vi "Map Tags to Channels.vi"(7 "instance id":string, 8 "error in (no error)":errorcluster, 9 "String Array":string[][](array[string]), 10 "Lines":T1[](array[typedef]), 11 "engine configuration in":refnum<class "engine configuration.lvclass">) -> (0 "error out":errorcluster, 3 "engine configuration out":refnum<class "engine configuration.lvclass">)   [LabVIEW 2015, in "PID Module editor node.lvclass"]
uses:
  PID Module editor node.lvclass
  module/configuration/Line.ctl
  <vilib>/NI/Tag Bus Module Framework/channel/TBM channel.lvclass
  <vilib>/NI/Module Execution Interface/Engine Configuration/engine configuration.lvclass
  <vilib>/NI/Tag Bus/tag/tag descriptor.lvclass/tag descriptor.ctl
  <vilib>/NI/Tag Bus/tag/tag descriptor.lvclass
  module/configuration/PID Module configuration.lvclass
panel:
  out "Numeric 2":i32
  out "Numeric":i32
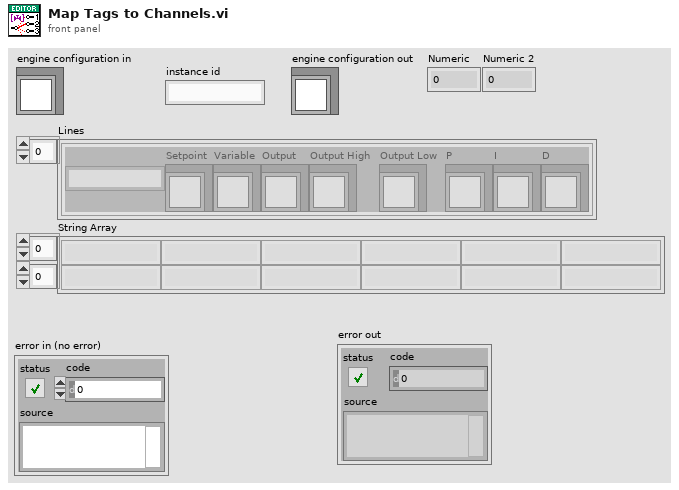
[diagram p1: front panel]
types:
  T1 = typedef "PID Module configuration.lvclass/Line.ctl" = cluster{"PID ID":string, "Setpoint":refnum<class "TBM channel.lvclass">, "Variable":refnum<class "TBM channel.lvclass">, "Output":refnum<class "TBM channel.lvclass">, "Output High":refnum<class "TBM channel.lvclass">, "Output Low":refnum<class "TBM channel.lvclass">, "P":refnum<class "TBM channel.lvclass">, "I":refnum<class "TBM channel.lvclass">, "D":refnum<class "TBM channel.lvclass">}
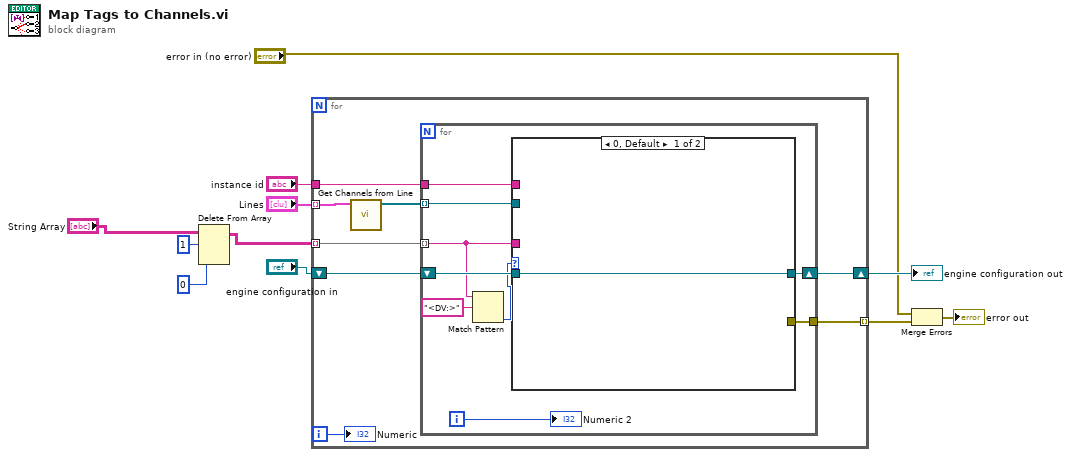
[diagram p0: block diagram]
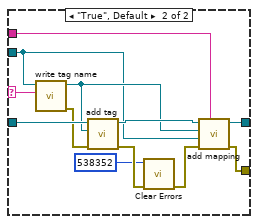
[diagram p3: hidden frame]
diagram:
  n1 = Delete From Array(array="String Array", length=1, index (col)=0 ("disabled index (col)")) -> (array with subset deleted=w1:string[][])  [unwired: 1 in, 1 out]
  n2 = for {
    tunnel: "Lines" -> [w14] mode=indexing
    tunnel: w1 -> [w15] mode=indexing
    shift-right: [w19] -> w8
    shift-left: "engine configuration in" -> [w16]
    tunnel: "instance id" -> [w18]
    tunnel: [w17] -> w10 mode=indexing
    i -> [w12]
    n3 = call "Get Channels from Line.vi"("Line"=w14) -> ("Channels"=w13:refnum<class "TBM channel.lvclass">[])  [unwired: 10 in]
    n4 = for {
      tunnel: w18 -> [w27]
      tunnel: [w26] -> w17
      tunnel: w13 -> [w24] mode=indexing
      tunnel: w15 -> [w22] mode=indexing
      shift-right: [w28] -> w19
      shift-left: w16 -> [w25]
      i -> [w23]
      n5 = Match Pattern(string=w22, regular expression="<DV:>") -> (offset past match=w20:i32)  [unwired: 1 in, 3 out]
      n6 = case shown="0, Default" w20 {
        tunnel: [w29 w35] -> w28
        tunnel: w27 -> [_ w34]
        tunnel: [_ w33] -> w26
        tunnel: w25 -> [w29 w32]
        tunnel: w24 -> [_ w31]
        tunnel: w22 -> [_ w30]
        frame 0, Default {
        }
        frame -1 {
          n7 = case shown="\"\"" w30 {
            selector: w30 -> [_ w37]
            tunnel: [w36 w48] -> w35
            tunnel: w34 -> [_ w47]
            tunnel: [_ w46] -> w33
            tunnel: w32 -> [w36 w45]
            tunnel: w31 -> [_ w42]
            frame "" {
            }
            frame "True", Default {
              n8 = call <vilib>:"write tag name.vi"("name"=w37, "system tag in"=w42) -> ("error out"=w41:errorcluster, "system tag out"=w43:refnum<class "TBM channel.lvclass">)  [unwired: 8 in]
              n9 = call-dynamic "add tag.vi"("error in"=w41, "tag descriptor"=w43, "engine configuration in"=w45) -> ("error out"=w40:errorcluster, "engine configuration out"=w44:refnum<class "engine configuration.lvclass">)  [unwired: 7 in]
              n10 = call <vilib>:"Clear Errors.vi"("error in (no error)"=w40, "specific error code to clear (0: all)"=538352) -> ("error out"=w39:errorcluster)  [unwired: 4 in, 1 out]
              n11 = call-dynamic "add mapping.vi"("owner ID"=w47, "error in"=w39, "channel"=w42, "tag descriptor"=w43, "engine configuration"=w44) -> ("error out"=w46:errorcluster, "engine configuration out"=w48:refnum<class "engine configuration.lvclass">)  [unwired: 5 in]
            }
          }
        }
      }
      "Numeric 2" <- w23
    }
    "Numeric" <- w12
  }
  "engine configuration out" <- w8
  n12 = Merge Errors("error in (no error)", w10) -> (→"error out":errorcluster)
